vi "Prcoess Converter.vi"(8 "error in":errorcluster, 11 "Fluidic Process in":string[][](array[string])) -> (0 "error out":errorcluster, 3 "Fluidic Process out":T1[](array[typedef]))   [LabVIEW 2019, in "Fluidic Process.lvlib"]
uses:
  Fluidic Process.lvlib
  Fluidic Data.ctl
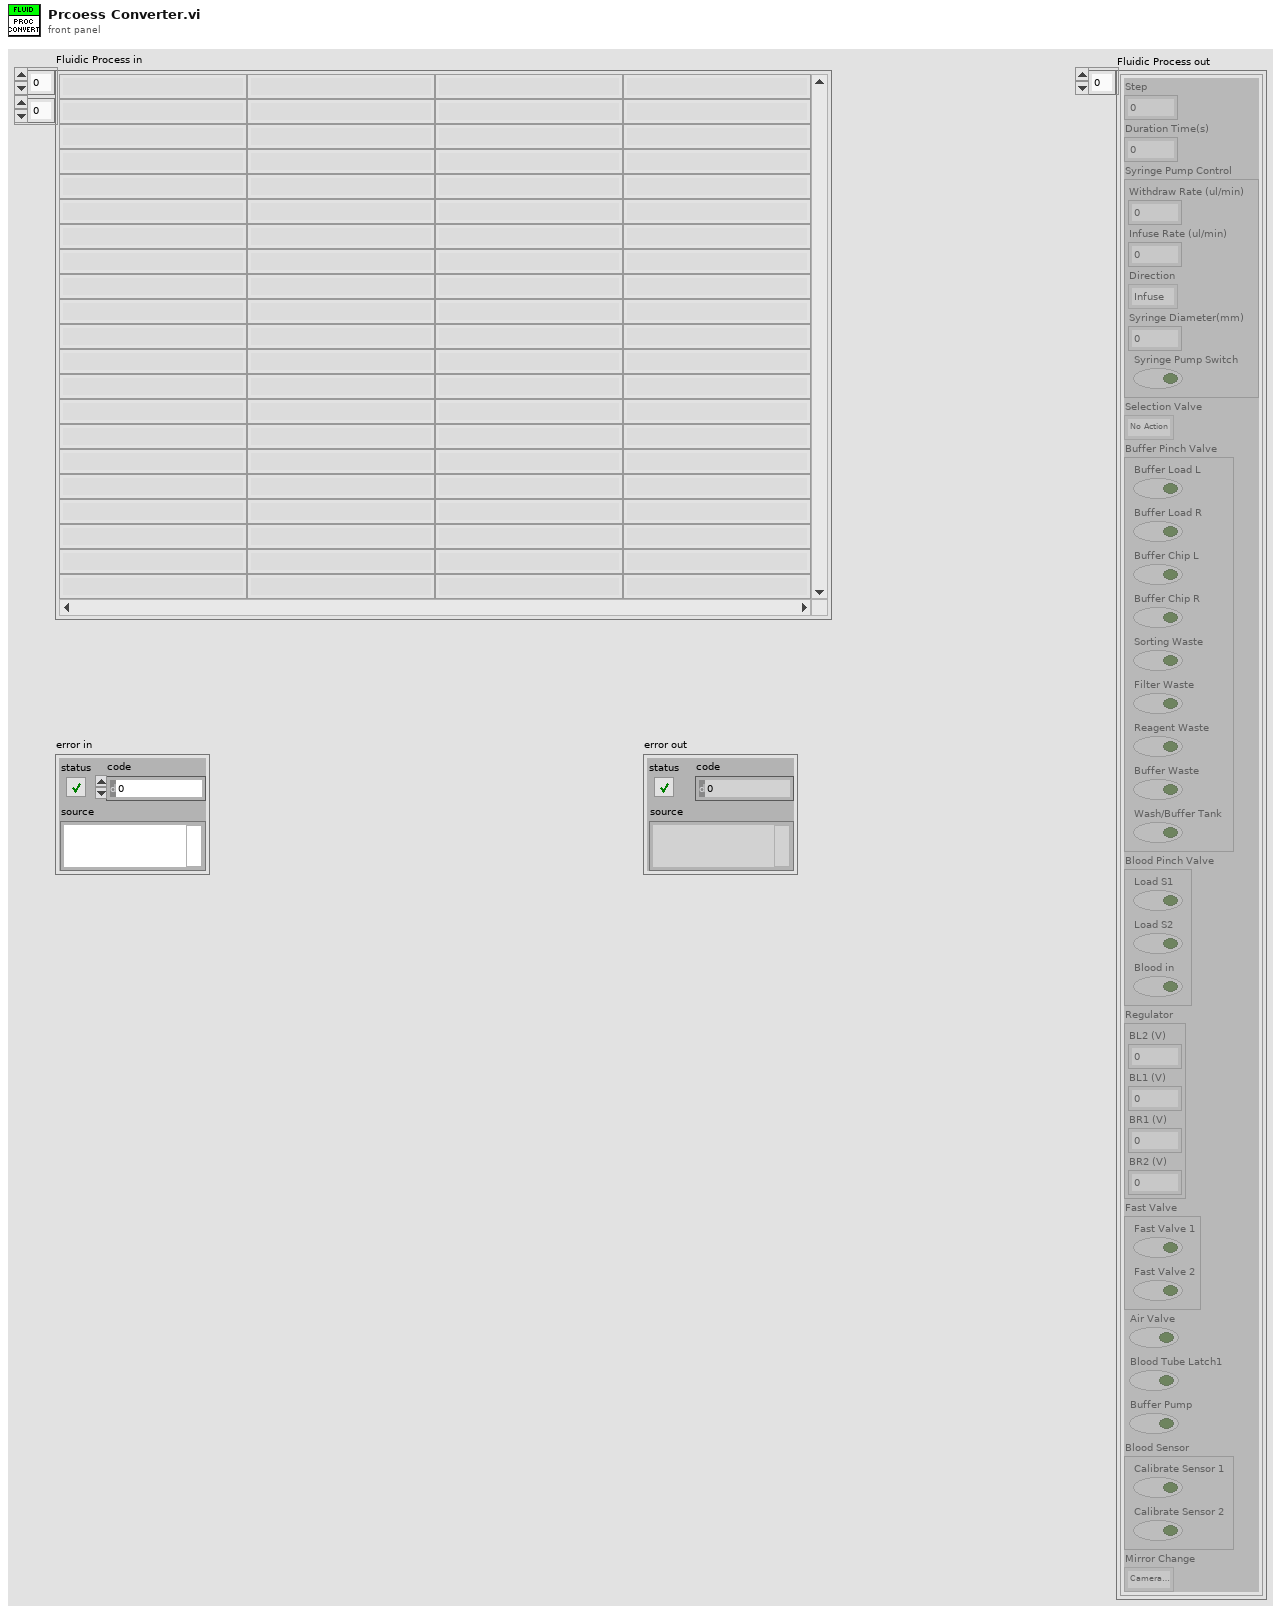
[diagram p1: front panel]
types:
  T1 = typedef "Fluidic Process.lvlib/Fluidic Data.ctl" = cluster{"Step":i32, "Duration Time(s)":i32, "Syringe Pump Control":cluster{"Withdraw Rate (ul/min)":dbl, "Infuse Rate (ul/min)":dbl, "Direction":enum16{"Infuse", "Withdraw"}, "Syringe Diameter(mm)":dbl, "Syringe Pump Switch":bool}, "Selection Valve":enum16{"No Action", "Position 1", "Position 2", "Position 3", "Position 4", "Position 5", "Position 6"}, "Buffer Pinch Valve":cluster{"Buffer Load L":bool, "Buffer Load R":bool, "Buffer Chip L":bool, "Buffer Chip R":bool, "Sorting Waste":bool, "Filter Waste":bool, "Reagent Waste":bool, "Buffer Waste":bool, "Wash/Buffer Tank":bool}, "Blood Pinch Valve":cluster{"Load S1":bool, "Load S2":bool, "Blood in":bool}, "Regulator":cluster{"BL2 (V)":fxp<+,16,3>, "BL1 (V)":fxp<+,16,3>, "BR1 (V)":fxp<+,16,3>, "BR2 (V)":fxp<+,16,3>}, "Fast Valve":cluster{"Fast Valve 1":bool, "Fast Valve 2":bool}, "Air Valve":bool, "Blood Tube Latch1":bool, "Buffer Pump":bool, "Blood Sensor":cluster{"Calibrate Sensor 1":bool, "Calibrate Sensor 2":bool}, "Mirror Change":enum16{"Camera Side", "SiPM Side"}}
  T2 = enum16{"No Action", "Position 1", "Position 2", "Position 3", "Position 4", "Position 5", "Position 6"}
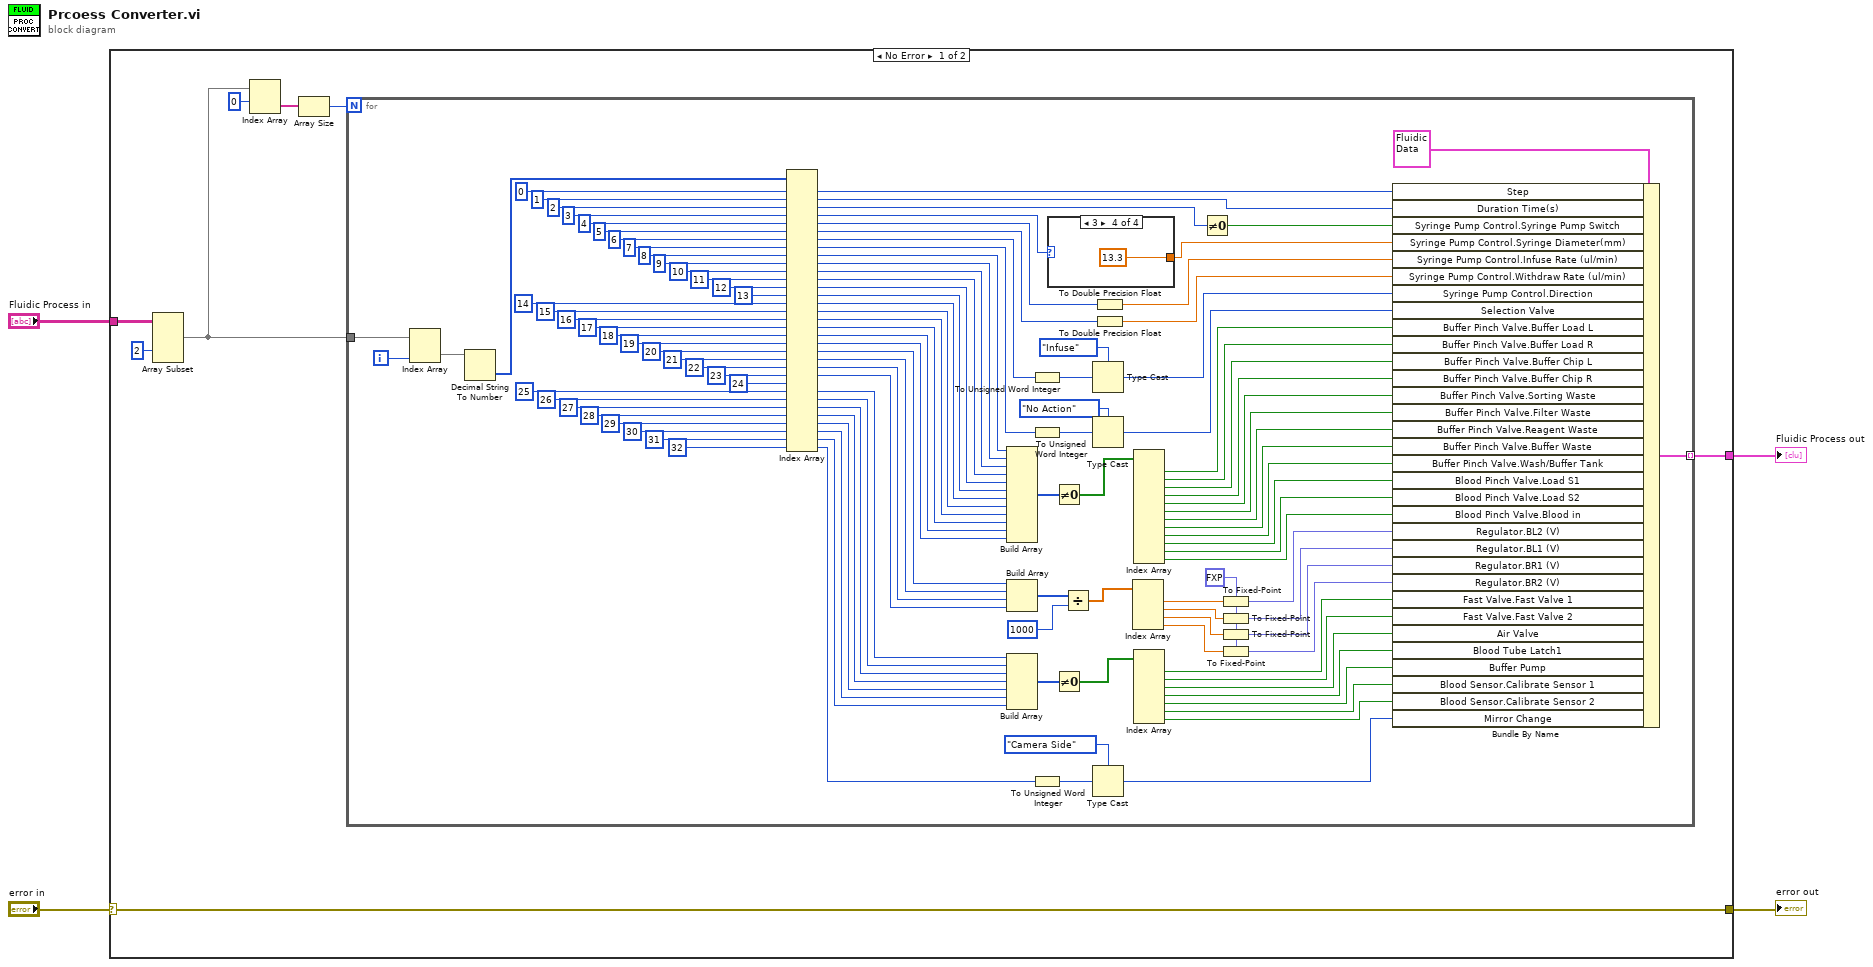
[diagram p0: block diagram]
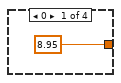
[diagram p2: hidden frame]
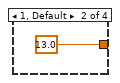
[diagram p3: hidden frame]
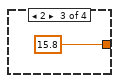
[diagram p4: hidden frame]
diagram:
  n1 = case shown="No Error" "error in" {
    selector: "error in" -> [w5 w136]
    tunnel: "Fluidic Process in" -> [w7 _]
    tunnel: [w6 _] -> w3
    tunnel: [w5 w136] -> w1
    frame No Error {
      n2 = Array Subset(array=w7, index (col)=2 ("index")) -> (w11:string[][])  [unwired: 3 in]
      n3 = Index Array(array=w11, index (row)=0) -> (element=w9:string[])  [unwired: 1 in]
      n4 = Array Size(array=w9) -> (size(s)=w8:i32)
      n5 = for {
        N: w8 -> [_]
        tunnel: w11 -> [w131]
        tunnel: [w75] -> w6 mode=indexing
        i -> [w130]
        w71 = fxp<+,16,3> 0.0 ("Regulator.BL2 (V)")
        n6 = Index Array(array=w131, index (col)=w130) -> (element=w128:string[])  [unwired: 1 in]
        n7 = Decimal String To Number(string=w128) -> (number=w127:i32[])  [unwired: 2 in, 1 out]
        n8 = Index Array(array=w127, index #1=0 ("index"), index #2=1 ("index"), index #3=2 ("index"), index #4=3 ("index"), index #5=4 ("index"), index #6=5 ("index"), index #7=6 ("index"), index #8=7 ("index"), index #9=8 ("index"), index #10=9 ("index"), index #11=10 ("index"), index #12=11 ("index"), index #13=12 ("index"), index #14=13 ("index"), index #15=14 ("index"), index #16=15 ("index"), index #17=16 ("index"), index #18=17 ("index"), index #19=18 ("index"), index #20=19 ("index"), index #21=20 ("index"), index #22=21 ("index"), index #23=22 ("index"), index #24=23 ("index"), index #25=24 ("index"), index #26=25 ("index"), index #27=26 ("index"), index #28=27 ("index"), index #29=28 ("index"), index #30=29 ("index"), index #31=30 ("index"), index #32=31 ("index"), index #33=32 ("index")) -> (element #1=w126:i32, element #2=w125:i32, element #3=w124:i32, element #4=w122:i32, element #5=w120:i32, element #6=w119:i32, element #7=w62:i32, element #8=w25:i32, element #9=w112:i32, element #10=w111:i32, element #11=w110:i32, element #12=w109:i32, element #13=w108:i32, element #14=w107:i32, element #15=w106:i32, element #16=w105:i32, element #17=w104:i32, element #18=w103:i32, element #19=w102:i32, element #20=w101:i32, element #21=w24:i32, element #22=w23:i32, element #23=w22:i32, element #24=w21:i32, element #26=w20:i32, element #27=w19:i32, element #28=w18:i32, element #29=w17:i32, element #30=w16:i32, element #31=w15:i32, element #32=w14:i32, element #33=w13:i32)  [unwired: 1 out]
        n9 = Build Array(w112, w111, w110, w109, w108, w107, w106, w105, w104, w103, w102, w101) -> (w100:i32[])
        n10 = Build Array(w24, w23, w22, w21) -> (w74:i32[])
        n11 = Build Array(w20, w19, w18, w17, w16, w15, w14) -> (w86:i32[])
        n12 = To Unsigned Word Integer(number=w62) -> (unsigned 16bit integer=w61:u16)
        n13 = To Unsigned Word Integer(number=w25) -> (unsigned 16bit integer=w60:u16)
        n14 = To Unsigned Word Integer(number=w13) -> (unsigned 16bit integer=w59:u16)
        n15 = case shown="3" w122 {
          tunnel: [8.95 13.0 15.8 13.3] -> w121
          frame 0 {
          }
          frame 1, Default {
          }
          frame 2 {
          }
          frame 3 {
          }
        }
        n16 = Not Equal To 0?(x=w100) -> (x != 0?=w99:bool[])
        n17 = Not Equal To 0?(x=w86) -> (x != 0?=w85:bool[])
        n18 = Divide(x=w74, y=1000) -> (x/y=w72:dbl[])
        n19 = Type Cast(type=enum16{"Infuse", "Withdraw"}."Infuse" ("Syringe Pump Control.Direction"), x=w61) -> (*(type *) &x=w115:enum16{"Infuse", "Withdraw"})
        n20 = Type Cast(type=T2."No Action" ("Selection Valve"), x=w60) -> (*(type *) &x=w113:T2)
        n21 = Type Cast(type=enum16{"Camera Side", "SiPM Side"}."Camera Side" ("Mirror Change"), x=w59) -> (*(type *) &x=w76:enum16{"Camera Side", "SiPM Side"})
        n22 = To Double Precision Float(number=w120) -> (double precision float=w118:dbl)
        n23 = To Double Precision Float(number=w119) -> (double precision float=w117:dbl)
        n24 = Index Array(array=w72) -> (element #1=w70:dbl, element #2=w69:dbl, element #3=w68:dbl, element #4=w67:dbl)  [unwired: 4 in]
        n25 = Index Array(array=w99) -> (element #1=w98:bool, element #2=w97:bool, element #3=w96:bool, element #4=w95:bool, element #5=w94:bool, element #6=w93:bool, element #7=w92:bool, element #8=w91:bool, element #9=w90:bool, element #10=w89:bool, element #11=w88:bool, element #12=w87:bool)  [unwired: 12 in]
        n26 = Index Array(array=w85) -> (element #1=w84:bool, element #2=w83:bool, element #3=w82:bool, element #4=w81:bool, element #5=w80:bool, element #6=w79:bool, element #7=w78:bool)  [unwired: 7 in]
        n27 = Not Equal To 0?(x=w124) -> (x != 0?=w123:bool)
        n28 = To Fixed-Point(fixed-point type=w71, number=w70) -> (fixed-point=w66:fxp<+,16,3>)
        n29 = To Fixed-Point(fixed-point type=w71, number=w69) -> (fixed-point=w65:fxp<+,16,3>)
        n30 = To Fixed-Point(fixed-point type=w71, number=w68) -> (fixed-point=w64:fxp<+,16,3>)
        n31 = To Fixed-Point(fixed-point type=w71, number=w67) -> (fixed-point=w63:fxp<+,16,3>)
        n32 = Bundle By Name(cluster=T1 {"Step"=0, "Duration Time(s)"=0, "Syringe Pump Control"={"Withdraw Rate (ul/min)"=0.0, "Infuse Rate (ul/min)"=0.0, "Direction"=enum."Infuse", "Syringe Diameter(mm)"=0.0, "Syringe Pump Switch"=FALSE}, "Selection Valve"=enum."No Action", "Buffer Pinch Valve"={"Buffer Load L"=FALSE, "Buffer Load R"=FALSE, "Buffer Chip L"=FALSE, "Buffer Chip R"=FALSE, "Sorting Waste"=FALSE, "Filter Waste"=FALSE, "Reagent Waste"=FALSE, "Buffer Waste"=FALSE, "Wash/Buffer Tank"=FALSE}, "Blood Pinch Valve"={"Load S1"=FALSE, "Load S2"=FALSE, "Blood in"=FALSE}, "Regulator"={"BL2 (V)"=0.0, "BL1 (V)"=0.0, "BR1 (V)"=0.0, "BR2 (V)"=0.0}, "Fast Valve"={"Fast Valve 1"=FALSE, "Fast Valve 2"=FALSE}, "Air Valve"=FALSE, "Blood Tube Latch1"=FALSE, "Buffer Pump"=FALSE, "Blood Sensor"={"Calibrate Sensor 1"=FALSE, "Calibrate Sensor 2"=FALSE}, "Mirror Change"=enum."Camera Side"} ("Cluster"), "Step"=w126, "Duration Time(s)"=w125, "Syringe Pump Control.Syringe Pump Switch"=w123, "Syringe Pump Control.Syringe Diameter(mm)"=w121, "Syringe Pump Control.Infuse Rate (ul/min)"=w118, "Syringe Pump Control.Withdraw Rate (ul/min)"=w117, "Syringe Pump Control.Direction"=w115, "Selection Valve"=w113, "Buffer Pinch Valve.Buffer Load L"=w98, "Buffer Pinch Valve.Buffer Load R"=w97, "Buffer Pinch Valve.Buffer Chip L"=w96, "Buffer Pinch Valve.Buffer Chip R"=w95, "Buffer Pinch Valve.Sorting Waste"=w94, "Buffer Pinch Valve.Filter Waste"=w93, "Buffer Pinch Valve.Reagent Waste"=w92, "Buffer Pinch Valve.Buffer Waste"=w91, "Buffer Pinch Valve.Wash/Buffer Tank"=w90, "Blood Pinch Valve.Load S1"=w89, "Blood Pinch Valve.Load S2"=w88, "Blood Pinch Valve.Blood in"=w87, "Regulator.BL2 (V)"=w66, "Regulator.BL1 (V)"=w65, "Regulator.BR1 (V)"=w64, "Regulator.BR2 (V)"=w63, "Fast Valve.Fast Valve 1"=w84, "Fast Valve.Fast Valve 2"=w83, "Air Valve"=w82, "Blood Tube Latch1"=w81, "Buffer Pump"=w80, "Blood Sensor.Calibrate Sensor 1"=w79, "Blood Sensor.Calibrate Sensor 2"=w78, "Mirror Change"=w76) -> (w75:T1)
      }
    }
    frame Error {
    }
  }
  "Fluidic Process out" <- w3
  "error out" <- w1
